vi "Keithley 2600 Series Generate Pulse With Voltage Protection Level.vi"() -> ()   [LabVIEW 2015]
doc: "This example demonstrates how to use the 2601B-PULSE pulser to generate a current pulse with a\nvoltage protection level"
uses:
  Keithley 2600 Series.lvlib
panel:
  out "Pulse Measurement":string
  out "Tripped Status":bool
  in  "Voltage Range (10V)":i32(ring)=1 items=["5", "10"]
  in  "Aperture(0.000001)":dbl=1e-05 format="%#_13g"
  in  "Delay(0)":dbl=3.5e-05 format="%#_13g"
  in  "Pulse Width(0 S)":dbl=5e-05 format="%#_13g"
  in  "Voltage Protection Level (20V)":dbl=8.0 format="%#_13g"
  in  "Current Range (10A)":i32(ring) items=["1", "5", "10", "0.250000"]
  in  "Trigger Count (1)":i32=1
  in  "VISA resource name":refnum<visa-resource-name>
  in  "Source Measure Unit Channel (0: Channel A)":i32(ring) items=["Channel A", "Channel B"]
  # "(c) 2020 - 2022 National Instruments.  ALL RIGHTS RESERVED."
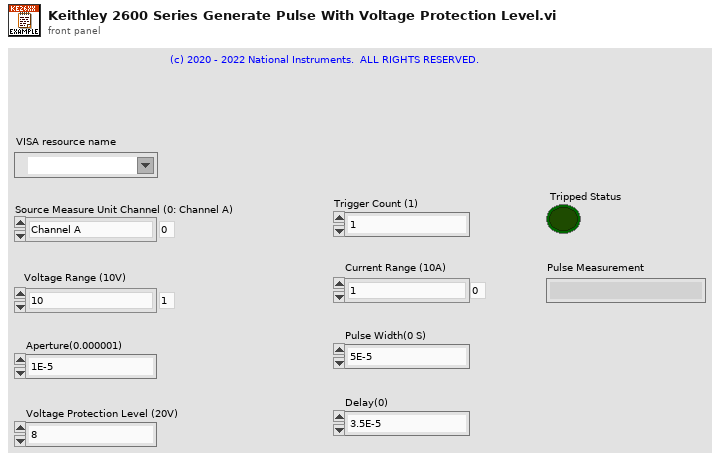
[diagram p1: front panel]
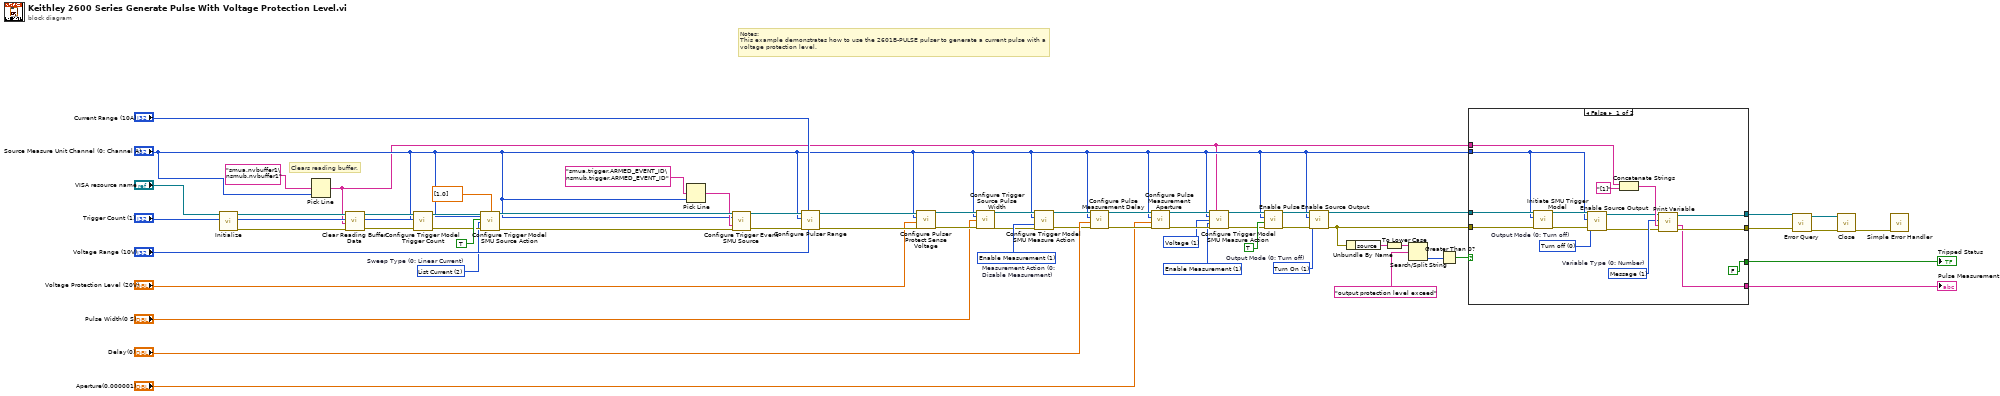
[diagram p0: block diagram]
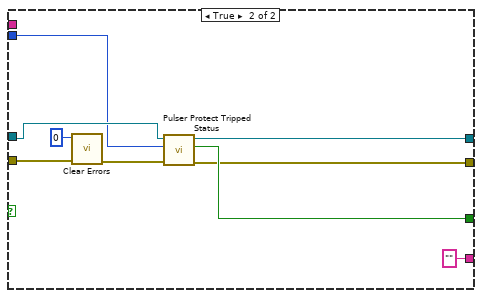
[diagram p2: hidden frame]
diagram:
  w12 = 1 items=["Disable Measurement", "Enable Measurement", "Enable Asynchronous Measurement "] ("Measurement Action (0: Disable Measurement)")
  w13 = 1 items=["Current", "Voltage", "Resistance", "Power", "Current and Voltage"] ("Measurement Type (0: Current)")
  w21 = 1 items=["Turn off", "Turn On", "High-Z"]  # Output Mode (0: Turn off)
  w24 = 2 items=["Linear Current", "Linear Voltage", "List Current", "List Voltage", "Logarithmic Current", "Logarithmic Voltage"]  # Sweep Type (0: Linear Current)
  w39 = 1 items=["Disable Measurement", "Enable Measurement", "Enable Asynchronous Measurement "]  # Measurement Action (0: Disable Measurement)
  # "Notes:\nThis example demonstrates how to use the 2601B-PULSE pulser to generate a current pulse with a\nvoltage protection level."
  # "Clears reading buffer."
  n1 = call "Initialize.vi"("VISA resource name"="VISA resource name") -> ("error out"=w59:errorcluster, "VISA resource name out"=w60:refnum<visa-resource-name>)  [unwired: 9 in]
  n2 = Pick Line(multi-line string="smua.nvbuffer1\nsmub.nvbuffer1", line index="Source Measure Unit Channel (0: Channel A)") -> (output string=w11:string)  [unwired: 1 in]
  n3 = call "Clear Reading Buffer Data.vi"("error in (no error)"=w59, "Reading Buffer (smua.nvbuffer1)"=w11, "VISA resource name"=w60) -> ("error out"=w56:errorcluster, "VISA resource name out"=w57:refnum<visa-resource-name>)  [unwired: 7 in]
  n4 = call "Configure Trigger Model Trigger Count.vi"("error in (no error)"=w56, "Trigger Count (1)"="Trigger Count (1)", "Source Measure Unit Channel (0: Channel A)"="Source Measure Unit Channel (0: Channel A)", "VISA resource name"=w57) -> ("error out"=w53:errorcluster, "VISA resource name out"=w55:refnum<visa-resource-name>)  [unwired: 6 in]
  n5 = call "Configure Trigger Model SMU Source Action.vi"("VISA resource name"=w55, "Source Measure Unit Channel (0: Channel A)"="Source Measure Unit Channel (0: Channel A)", "Enable Source Sweep (F: Disable)"=TRUE, "Sweep Type (0: Linear Current)"=w24, "error in (no error)"=w53, "Sweep List"=dbl[] [1.0]) -> ("VISA resource name out"=w52:refnum<visa-resource-name>, "error out"=w51:errorcluster)  [unwired: 12 in]
  n6 = Pick Line(multi-line string="smua.trigger.ARMED_EVENT_ID\nsmub.trigger.ARMED_EVENT_ID", line index="Source Measure Unit Channel (0: Channel A)") -> (output string=w49:string)  [unwired: 1 in]
  n7 = call "Configure Trigger Event SMU Source.vi"("VISA resource name"=w52, "Source Measure Unit Channel (0: Channel A)"="Source Measure Unit Channel (0: Channel A)", "Event ID"=w49, "error in (no error)"=w51) -> ("VISA resource name out"=w48:refnum<visa-resource-name>, "error out"=w47:errorcluster)  [unwired: 10 in]
  n8 = call "Configure Pulser Range.vi"("Voltage Range (10V)"="Voltage Range (10V)", "Current Range (10A)"="Current Range (10A)", "error in (no error)"=w47, "Source Measure Unit Channel (0: Channel A)"="Source Measure Unit Channel (0: Channel A)", "VISA resource name"=w48) -> ("error out"=w45:errorcluster, "VISA resource name out"=w46:refnum<visa-resource-name>)  [unwired: 5 in]
  n9 = call "Configure Pulser Protect Sense Voltage.vi"("error in (no error)"=w45, "Voltage Protection Level (20V)"="Voltage Protection Level (20V)", "Source Measure Unit Channel (0: Channel A)"="Source Measure Unit Channel (0: Channel A)", "VISA resource name"=w46) -> ("error out"=w42:errorcluster, "VISA resource name out"=w43:refnum<visa-resource-name>)  [unwired: 6 in]
  n10 = call "Configure Trigger Source Pulse Width.vi"("VISA resource name"=w43, "Source Measure Unit Channel (0: Channel A)"="Source Measure Unit Channel (0: Channel A)", "Pulse Width(0 S)"="Pulse Width(0 S)", "error in (no error)"=w42) -> ("VISA resource name out"=w40:refnum<visa-resource-name>, "error out"=w38:errorcluster)  [unwired: 10 in]
  n11 = call "Configure Trigger Model SMU Measure Action.vi"("VISA resource name"=w40, "Source Measure Unit Channel (0: Channel A)"="Source Measure Unit Channel (0: Channel A)", "Measurement Action (0: Disable Measurement)"=w39, "error in (no error)"=w38) -> ("VISA resource name out"=w37:refnum<visa-resource-name>, "error out"=w35:errorcluster)  [unwired: 10 in]
  n12 = call "Configure Pulse Measurement Delay.vi"("error in (no error)"=w35, "Delay(0)"="Delay(0)", "Source Measure Unit Channel (0: Channel A)"="Source Measure Unit Channel (0: Channel A)", "VISA resource name"=w37) -> ("error out"=w33:errorcluster, "VISA resource name out"=w34:refnum<visa-resource-name>)  [unwired: 6 in]
  n13 = call "Configure Pulse Measurement Aperture.vi"("error in (no error)"=w33, "Aperture(0.000001)"="Aperture(0.000001)", "Source Measure Unit Channel (0: Channel A)"="Source Measure Unit Channel (0: Channel A)", "VISA resource name"=w34) -> ("error out"=w15:errorcluster, "VISA resource name out"=w18:refnum<visa-resource-name>)  [unwired: 6 in]
  n14 = call "Configure Trigger Model SMU Measure Action.vi"("VISA resource name"=w18, "Reading Buffer 1 (smua.nvbuffer1)"=w11, "Source Measure Unit Channel (0: Channel A)"="Source Measure Unit Channel (0: Channel A)", "Measurement Type (0: Current)"=w13, "Measurement Action (0: Disable Measurement)"=w12, "error in (no error)"=w15) -> ("VISA resource name out"=w17:refnum<visa-resource-name>, "error out"=w16:errorcluster)  [unwired: 8 in]
  n15 = call "Enable Pulse.vi"("error in (no error)"=w16, "Enable Pulser (Enable)"=TRUE, "Source Measure Unit Channel (0: Channel A)"="Source Measure Unit Channel (0: Channel A)", "VISA resource name"=w17) -> ("error out"=w20:errorcluster, "VISA resource name out"=w22:refnum<visa-resource-name>)  [unwired: 6 in]
  n16 = call "Enable Source Output.vi"("error in (no error)"=w20, "Output Mode (0: Turn off)"=w21, "Source Measure Unit Channel (0: Channel A)"="Source Measure Unit Channel (0: Channel A)", "VISA resource name"=w22) -> ("error out"=w6:errorcluster, "VISA resource name out"=w19:refnum<visa-resource-name>)  [unwired: 6 in]
  n17 = Unbundle By Name(w6) -> ("source"=w8:string)
  n18 = To Lower Case(string=w8) -> (all lower case string=w7:string)
  n19 = Search/Split String(string=w7, search string/char (-)="output protection level exceed") -> (offset of match=w9:i32)  [unwired: 1 in, 2 out]
  n20 = Greater Than 0?(x=w9) -> (x > 0?=w5:bool)
  n21 = case shown="False" w5 {
    tunnel: w6 -> [w77 w86]
    tunnel: w19 -> [w76 w83]
    tunnel: "Source Measure Unit Channel (0: Channel A)" -> [w71 w82]
    tunnel: w11 -> [w70 _]
    tunnel: [FALSE ("Tripped Status") w81] -> w4
    tunnel: [w64 w80] -> w1
    tunnel: [w63 w79] -> w2
    tunnel: [w62 "" ("Message")] -> w3
    frame False {
      w68 = 1 items=["Number", "Message"]  # Variable Type (0: Number)
      w74 = 0 items=["Turn off", "Turn On", "High-Z"]  # Output Mode (0: Turn off)
      n22 = call "Initiate SMU Trigger Model.vi"("error in (no error)"=w77, "Source Measure Unit Channel (0: Channel A)"=w71, "VISA resource name"=w76) -> ("error out"=w73:errorcluster, "VISA resource name out"=w75:refnum<visa-resource-name>)  [unwired: 7 in]
      n23 = call "Enable Source Output.vi"("error in (no error)"=w73, "Output Mode (0: Turn off)"=w74, "Source Measure Unit Channel (0: Channel A)"=w71, "VISA resource name"=w75) -> ("error out"=w66:errorcluster, "VISA resource name out"=w67:refnum<visa-resource-name>)  [unwired: 6 in]
      n24 = Concatenate Strings(w70, "[1]" ("string")) -> (w69:string)
      n25 = call "Print Variable.vi"("error in (no error)"=w66, "Variable Name"=w69, "Variable Type (0: Number)"=w68, "VISA resource name"=w67) -> ("error out"=w63:errorcluster, "Message"=w62:string, "VISA resource name out"=w64:refnum<visa-resource-name>)  [unwired: 4 in, 1 out]
    }
    frame True {
      n26 = call <vilib>:"Clear Errors.vi"("error in (no error)"=w86, "specific error code to clear (0: all)"=0) -> ("error out"=w84:errorcluster)  [unwired: 4 in, 1 out]
      n27 = call "Pulser Protect Tripped Status.vi"("error in (no error)"=w84, "Source Measure Unit Channel (0: Channel A)"=w82, "VISA resource name"=w83) -> ("error out"=w79:errorcluster, "Tripped Status"=w81:bool, "VISA resource name out"=w80:refnum<visa-resource-name>)  [unwired: 6 in]
    }
  }
  "Tripped Status" <- w4
  "Pulse Measurement" <- w3
  n28 = call "Error Query.vi"("error in (no error)"=w2, "VISA resource name"=w1) -> ("error out"=w31:errorcluster, "VISA resource name out"=w30:refnum<visa-resource-name>)  [unwired: 6 in, 2 out]
  n29 = call "Close.vi"("error in (no error)"=w31, "VISA resource name"=w30) -> ("error out"=w29:errorcluster)  [unwired: 9 in]
  n30 = call <vilib>:"Simple Error Handler.vi"("error in (no error)"=w29) -> ()  [unwired: 4 in, 5 out]
